vi "HA2_yufan_dong.vi"(4 "Stop":bool, 5 "Save":bool, 6 "Measure":bool, 7 "File Path":path, 8 "Error In":errorcluster, 10 "Output Channel (LEDs)":tag="Dev1/port0/line0:1", 11 "Input Channel (AI)":tag="Dev1/ai0") -> (0 "Error Out":errorcluster, 2 "Average Chart":cluster{dbl, dbl}(graph), 3 "Waveform Chart":cluster{dbl, dbl}(graph))   [LabVIEW 2019]
doc: "This is a traffic light system. It realized the output with hard device or simulated device. The light has four phases."
uses:
  States_yufan_dong.ctl
  <vilib>/DAQmx/read.llb/DAQmx Read (Analog 1D DBL NChan 1Samp).vi
  <vilib>/DAQmx/write.llb/DAQmx Write (Digital 1D Bool 1Chan 1Samp).vi
  <vilib>/DAQmx/create/channels.llb/DAQmx Create Channel (DO-Digital Output).vi
  <vilib>/DAQmx/create/channels.llb/DAQmx Create Channel (AI-Voltage-Basic).vi
  <vilib>/DAQmx/configure/timing.llb/DAQmx Timing (Sample Clock).vi
  <vilib>/DAQmx/miscellaneous.llb/DAQmx Fill In Error Info.vi
  <resource>/objmgr/daqmx.rc
panel:
  out "Delay (ms)":u32
  out "Sample Rate (Hz)":dbl=50.0
  out "Meldung":string
  out "Red":bool
  out "Yellow":bool
  out "Green":bool
  # "Note & Guide\n\n<<<<<< Channels >>>>>\n\nInput Channel\n<device>/ai0:1\nmyDAQ1/ai0:1\n\nOutput Channel\n<device>/<port>/line0:2\nmyDAQ1/port0/line0:2\n\n\n\n<<<<<< Controls >>>>>\n\nStart and Pause\n\nStop\n\nSave Path\ncan create new document\ncan not create new folder\nnot existing folder = error\n\nSave\nstop measurement and save\n\n\n\n<<<<<<< Others >>>>>>\n\nSample Rate (Hz)\n50 as constant\nDelay (ms)\n~=20\n\nAuthor\nYufan Dong - 12.Oct.2021"
  # "Messprogramm"
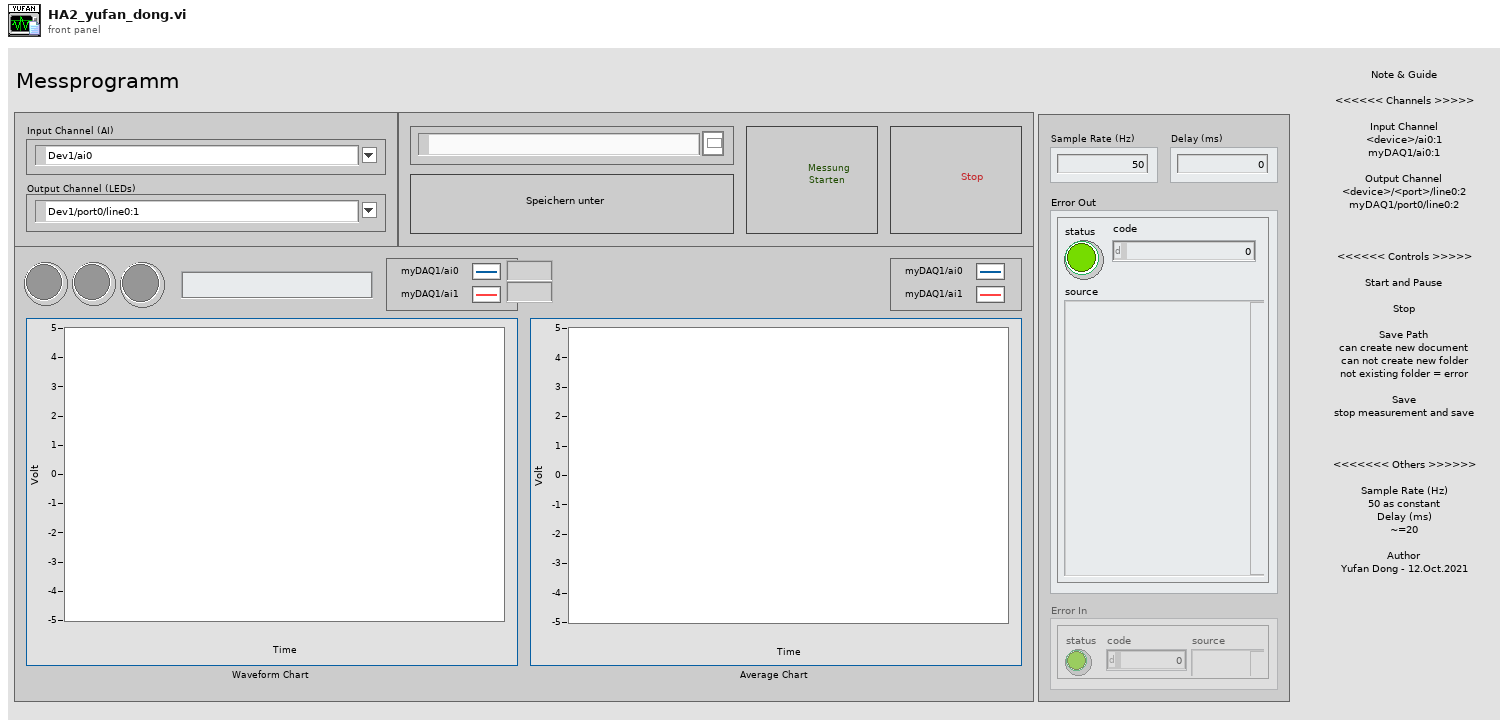
[diagram p1: front panel]
types:
  T1 = typedef "States_yufan_dong.ctl" = enum16{"pause", "measure", "save", "stop"}
  T2 = enum16{"open", "replace", "create", "open or create", "replace or create", "replace or create with confirmation"}
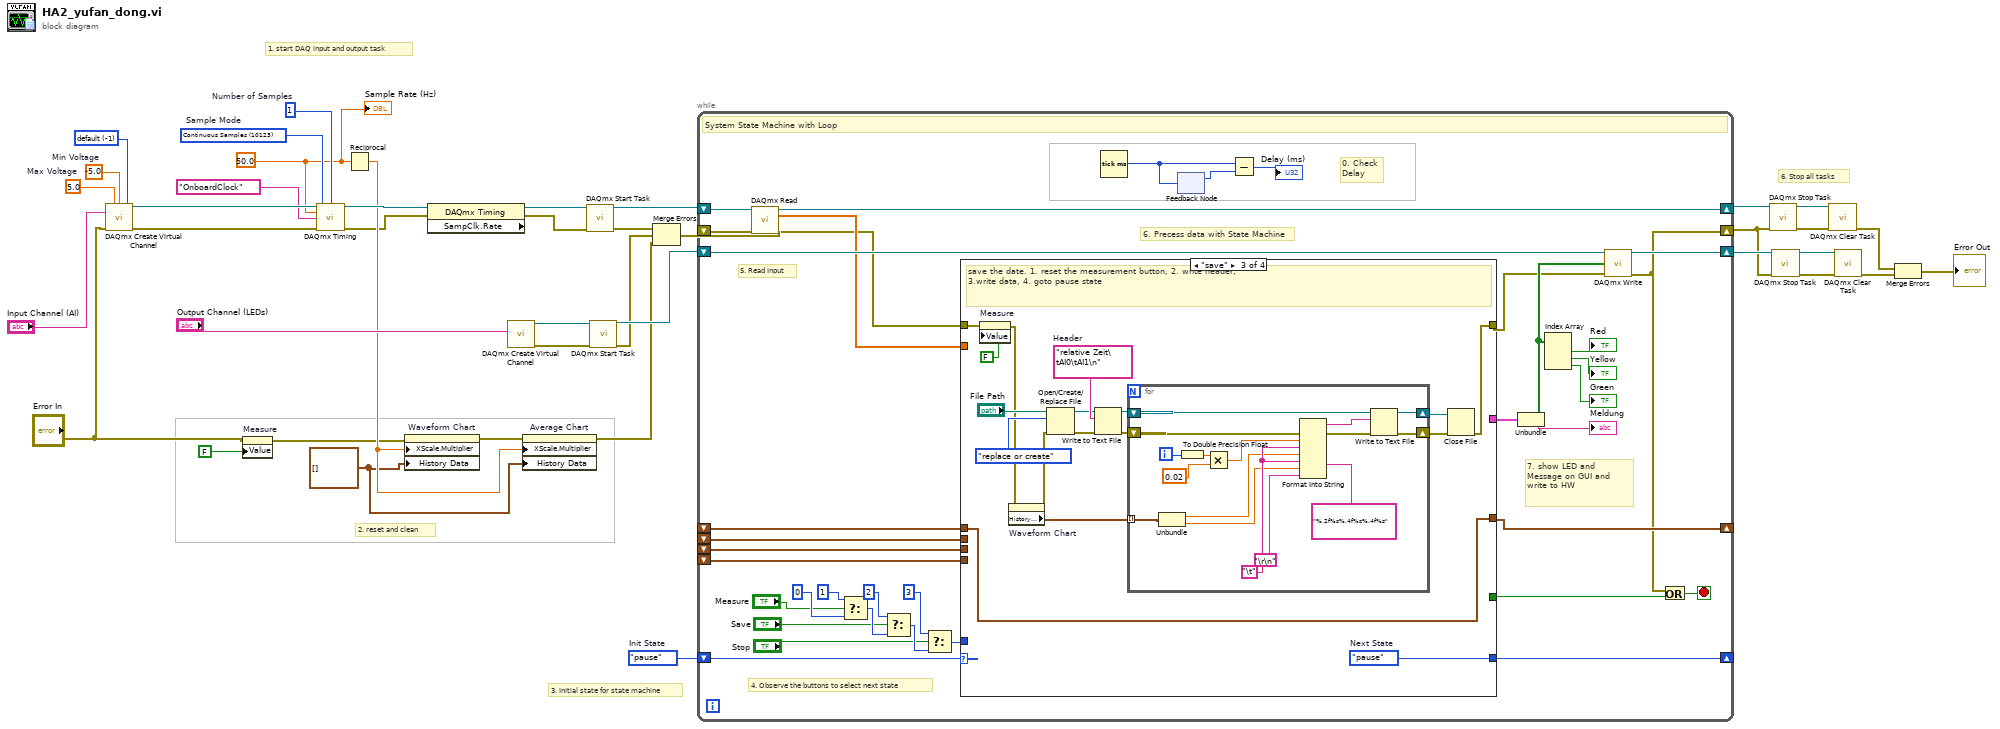
[diagram p0: block diagram]
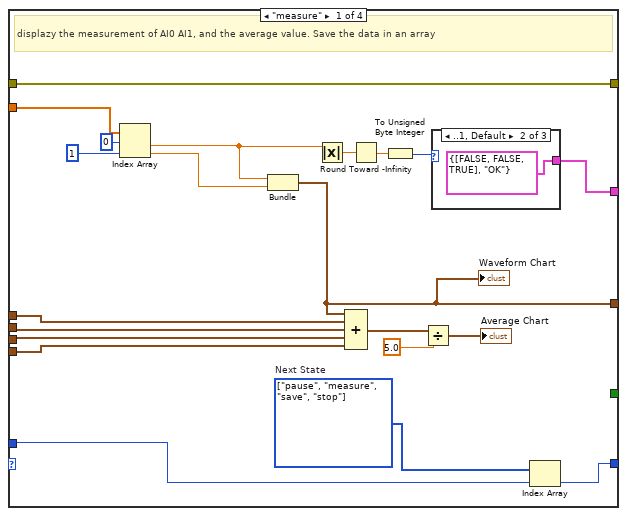
[diagram p2: hidden frame]
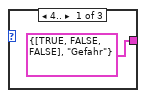
[diagram p3: hidden frame]
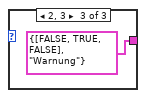
[diagram p4: hidden frame]
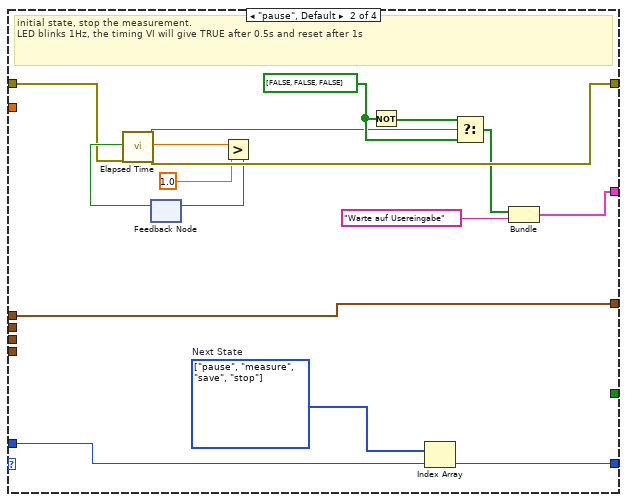
[diagram p5: hidden frame]
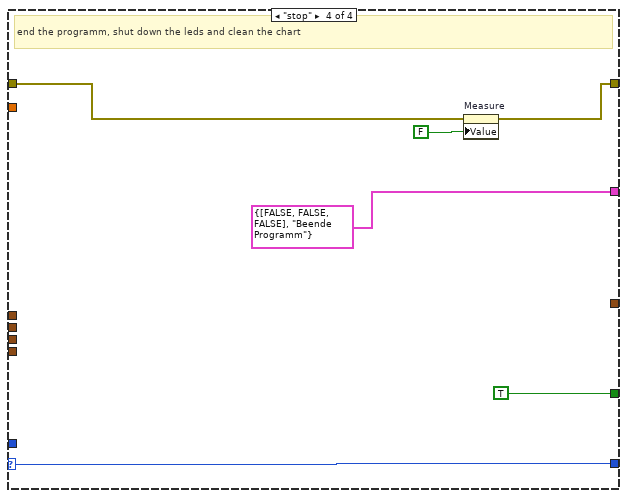
[diagram p6: hidden frame]
diagram:
  w5 = cluster{dbl, dbl}[] [] ("History Data")
  w21 = 50.0 ("Sample Rate")
  w26 = -1 items=["default"=-1, "RSE"=10083, "NRSE"=10078, "Differential"=10106, "Pseudodifferential"=12529] ("Terminal Configuration")
  w10 = States_yufan_dong."pause"  # Init State
  w29 = 1  # Number of Samples
  w30 = 5.0  # Max Voltage
  w31 = -5.0  # Min Voltage
  w36 = 10123 items=["Finite Samples"=10178, "Continuous Samples"=10123, "Hardware Timed Single Point"=12522]  # Sample Mode
  # "6. Stop all tasks"
  # "3. Initial state for state machine"
  # "1. start DAQ input and output task"
  # "2. reset and clean"
  n1 = call-poly <vilib>:"DAQmx Create Virtual Channel.vi"("maximum value"=w30, "minimum value"=w31, "input terminal configuration"=w26, "physical channels"="Input Channel (AI)", "error in"="Error In") -> ("task out"=w34:refnum<k21>, "error out"=w35:errorcluster)  [unwired: 9 in]
  n2 = property on="Measure" class="Bool (strict)"(error in="Error In", "Value"=FALSE) -> (error out=w2:errorcluster)  [unwired: 1 in, 1 out]
  n3 = call-poly <vilib>:"DAQmx Timing.vi"("task/channels in"=w34, "sample mode"=w36, "samples per channel"=w29, "rate"=w21, "source"=tag "OnboardClock" ("Sample Clock Source"), "error in"=w35) -> ("task out"=w37:refnum<k21>, "error out"=w7:errorcluster)  [unwired: 8 in]
  n4 = Reciprocal(x=w21) -> (1/x=w9:dbl)
  n5 = property on="Waveform Chart" class="WFChart (strict)"(error in=w2, "XScale.Multiplier"=w9, "History Data"=w5) -> (error out=w8:errorcluster)  [unwired: 1 in, 1 out]
  n6 = property class="DAQmx Timing" props=["SampClk.Rate"](reference=w37, error in=w7) -> (reference out=w18:refnum<k21>, error out=w17:errorcluster)  [unwired: 1 out]
  n7 = call-poly <vilib>:"DAQmx Create Virtual Channel.vi"("lines"="Output Channel (LEDs)") -> ("task out"=w38:refnum<k21>, "error out"=w39:errorcluster)  [unwired: 13 in]
  n8 = property on="Average Chart" class="WFChart (strict)"(error in=w8, "XScale.Multiplier"=w9, "History Data"=w5) -> (error out=w6:errorcluster)  [unwired: 1 in, 1 out]
  n9 = call <vilib>:"DAQmx Start Task.vi"("task/channels in"=w18, "error in"=w17) -> ("task out"=w33:refnum<k21>, "error out"=w16:errorcluster)  [unwired: 12 in]
  n10 = call <vilib>:"DAQmx Start Task.vi"("task/channels in"=w38, "error in"=w39) -> ("task out"=w24:refnum<k21>, "error out"=w15:errorcluster)  [unwired: 12 in]
  n11 = Merge Errors(w16, w15, w6) -> (w14:errorcluster)
  n12 = while {
    shift-right: [w60] -> w20
    shift-left: w33 -> [w66]
    shift-right: [w76] -> w19
    shift-left: w24 -> [w77]
    shift-right: [w41] -> w13
    shift-left: w14 -> [w65]
    shift-right: [w52] -> _
    shift-left: _ -> [w64]
    shift-left: _ -> [w63]
    shift-left: _ -> [w62]
    shift-left: _ -> [w61]
    shift-right: [w53] -> _
    shift-left: w10 -> [w57]
    stop <- w72 stop-if-true
    # "6. Precess data with State Machine"
    # "5. Read Input"
    # "7. show LED and Message on GUI and write to HW"
    # "4. Observe the buttons to select next state"
    # "0. Check \nDelay"
    # "System State Machine with Loop"
    n13 = call-poly <vilib>:"DAQmx Read.vi"("task/channels in"=w66, "error in"=w65) -> ("task out"=w60:refnum<k21>, "data"=w59:dbl[], "error out"=w58:errorcluster)  [unwired: 11 in]
    n14 = Select(t=1, s="Measure", f=0) -> (s? t:f=w50:i32)
    n15 = Select(t=2, s="Save", f=w50) -> (s? t:f=w51:i32)
    n16 = Select(t=3, s="Stop", f=w51) -> (s? t:f=w45:i32)
    n17 = case shown="\"save\"" w57 {
      selector: w57 -> [_ _ _ w154]
      tunnel: [w94 w107 _ cluster{bool[], string} {[FALSE, FALSE, FALSE], "Beende Programm"}] -> w56
      tunnel: [w83 w114 w124 w153] -> w55
      tunnel: w58 -> [w83 w106 w133 w151]
      tunnel: [w79 w103 w122 _] -> w52
      tunnel: w64 -> [w90 w103 w122 _]
      tunnel: w63 -> [w89 _ _ _]
      tunnel: w62 -> [w88 _ _ _]
      tunnel: w61 -> [w87 _ _ _]
      tunnel: w59 -> [w78 _ _ _]
      tunnel: [_ _ _ TRUE] -> w54
      tunnel: [w81 w105 w123 w154] -> w53
      tunnel: w45 -> [w80 w104 _ _]
      frame "measure" {
        w82 = T1[] [enum."pause", enum."measure", enum."save", enum."stop"] items=["pause", "measure", "save", "stop"]  # Next State
        # "displazy the measurement of AI0 AI1, and the average value. Save the data in an array"
        n18 = Index Array(array=w78, index #1=0, index #2=1) -> (element #1=w92:dbl, element #2=w91:dbl)
        n19 = Bundle("Waveform"=w92, "Waveform"=w91) -> (w79:cluster{"Waveform":dbl, "Waveform":dbl})  [unwired: 1 in]
        "Waveform Chart" <- w79
        n20 = Absolute Value(x=w92) -> (abs(x)=w96:dbl)
        n21 = Compound Arithmetic op=ADD(w79, w90, w89, w88, w87) -> (w86:cluster{"Waveform":dbl, "Waveform":dbl})
        n22 = Round Toward -Infinity(1:w96) -> (0:w98:dbl)
        n23 = To Unsigned Byte Integer(number=w98) -> (unsigned 8bit integer=w97:u8)
        n24 = Divide(x=w86, y=5.0) -> (x/y=→"Average Chart":cluster{"Waveform":dbl, "Waveform":dbl})
        n25 = case shown="..1, Default" w97 {
          tunnel: [cluster{bool[], string} {[TRUE, FALSE, FALSE], "Gefahr"} cluster{bool[], string} {[FALSE, FALSE, TRUE], "OK"} cluster{bool[], string} {[FALSE, TRUE, FALSE], "Warnung"}] -> w94
          frame 4.. {
          }
          frame ..1, Default {
          }
          frame 2, 3 {
          }
        }
        n26 = Index Array(array=w82, index=w80) -> (element=w81:T1)
      }
      frame "pause", Default {
        w102 = T1[] [enum."pause", enum."measure", enum."save", enum."stop"] items=["pause", "measure", "save", "stop"]  # Next State
        w117 = bool[] [FALSE, FALSE, FALSE]
        # "initial state, stop the measurement.\nLED blinks 1Hz, the timing VI will give TRUE after 0.5s and reset after 1s"
        n27 = feedback #1() -> (w110:bool)  [unwired: 1 in]
        n28 = call "Elapsed Time"("Reset"=w110, "error in (no error)"=w106) -> ("Elapsed Time (s)"=w112:dbl, "Time has Elapsed"=w116:bool, "error out"=w114:errorcluster)  [unwired: 10 in, 5 out]
        n29 = Greater?(x=w112, y=1.0) -> (0:w111:bool)
        n30 = feedback-in #1(w111) -> ()
        n31 = Not(x=w117) -> (.not. x?=w115:bool[])
        n32 = Index Array(array=w102, index=w104) -> (element=w105:T1)
        n33 = Select(t=w115, s=w116, f=w117) -> (s? t:f=w109:bool[])
        n34 = Bundle(w109, "Warte auf Usereingabe") -> (w107:cluster{bool[], string})  [unwired: 1 in]
      }
      frame "save" {
        w123 = States_yufan_dong."pause"  # Next State
        w130 = "relative Zeit\tAI0\tAI1\n"  # Header
        # "save the date. 1. reset the measurement button, 2. write header, \n3.write data, 4. goto pause state"
        n35 = property on="Measure" class="Bool (strict)"(error in=w133, "Value"=FALSE) -> (error out=w119:errorcluster)  [unwired: 1 in, 1 out]
        n36 = property on="Waveform Chart" class="WFChart (strict)"(error in=w119) -> (error out=w118:errorcluster, "History Data"=w121:cluster{dbl, dbl}[])  [unwired: 1 in, 1 out]
        n37 = Open/Create/Replace File(file path (use dialog)="File Path", error in=w118, operation (0:open)=T2."replace or create") -> (refnum out=w129:refnum<file>, error out=w120:errorcluster)  [unwired: 3 in, 1 out]
        n38 = Write to Text File(file (use dialog)=w129, text=w130, error in=w120) -> (refnum out=w127:refnum<file>, error out=w128:errorcluster)  [unwired: 1 in, 1 out]
        n39 = for {
          shift-right: [w139] -> w126
          shift-left: w128 -> [w142]
          shift-right: [w138] -> w125
          shift-left: w127 -> [w141]
          tunnel: w121 -> [w137] mode=indexing
          i -> [w150]
          w146 = "\t"
          n40 = Unbundle(w137) -> (w136:dbl, w135:dbl)
          n41 = To Double Precision Float(number=w150) -> (double precision float=w147:dbl)
          n42 = Multiply(x=w147, y=0.02) -> (x*y=w148:dbl)
          n43 = Format Into String(format string="%.2f%s%.4f%s%.4f%s", error in=w142, w148, w146, w136, w146, w135, "\r\n") -> (resulting string=w144:string, error out=w140:errorcluster)  [unwired: 1 in]
          n44 = Write to Text File(file (use dialog)=w141, text=w144, error in=w140) -> (refnum out=w138:refnum<file>, error out=w139:errorcluster)  [unwired: 1 in, 1 out]
        }
        n45 = Close File(refnum=w125, error in=w126) -> (error out=w124:errorcluster)  [unwired: 1 out]
      }
      frame "stop" {
        # "end the programm, shut down the leds and clean the chart"
        n46 = property on="Measure" class="Bool (strict)"(error in=w151, "Value"=FALSE) -> (error out=w153:errorcluster)  [unwired: 1 in, 1 out]
      }
    }
    n47 = Tick Count (ms)() -> (millisecond timer value=w74:u32)
    n48 = feedback #2() -> (w75:u32)  [unwired: 1 in]
    n49 = feedback-in #2(w74) -> ()
    n50 = Subtract(x=w74, y=w75) -> (x-y=→"Delay (ms)":u32)
    n51 = Unbundle(w56) -> (w67:bool[], →"Meldung":string)
    n52 = Index Array(array=w67) -> (element #1=→"Red":bool, element #2=→"Yellow":bool, element #3=→"Green":bool)  [unwired: 3 in]
    n53 = call-poly <vilib>:"DAQmx Write.vi"("task/channels in"=w77, "data"=w67, "error in"=w55) -> ("task out"=w76:refnum<k21>, "error out"=w41:errorcluster)  [unwired: 10 in, 1 out]
    n54 = Or(x=w41, y=w54) -> (x .or. y?=w72:bool)
  }
  n55 = call <vilib>:"DAQmx Stop Task.vi"("task/channels in"=w20, "error in"=w13) -> ("task out"=w27:refnum<k21>, "error out"=w28:errorcluster)  [unwired: 12 in]
  n56 = call <vilib>:"DAQmx Stop Task.vi"("task/channels in"=w19, "error in"=w13) -> ("task out"=w23:refnum<k21>, "error out"=w22:errorcluster)  [unwired: 12 in]
  n57 = call <vilib>:"DAQmx Clear Task.vi"("task in"=w27, "error in"=w28) -> ("error out"=w12:errorcluster)  [unwired: 13 in]
  n58 = call <vilib>:"DAQmx Clear Task.vi"("task in"=w23, "error in"=w22) -> ("error out"=w11:errorcluster)  [unwired: 13 in]
  n59 = Merge Errors(w12, w11) -> (→"Error Out":errorcluster)
  "Sample Rate (Hz)" <- w21
